vi "NT4 Prepare Tree Entries.vi"(11 "Topic List":T3(array[cluster]) {"NT_Type" items=["NT_Unassigned"=0, "NT_Boolean"=1, "NT_Double"=2, "NT_String"=4, "NT_Raw"=8, "NT_BooleanArray"=16, "NT_DoubleArray"=32, "NT_StringArray"=64, "NT_RPC"=128, "NT_Integer"=256, "NT_Float"=512, "NT_IntegerArray"=1024, "NT_FloatArray"=2048]}) -> (2 "Tokens":string[](array[string]), 3 "Sorted Tree Rows":T2(array[cluster]) {"NT_Type" items=["NT_Unassigned"=0, "NT_Boolean"=1, "NT_Double"=2, "NT_String"=4, "NT_Raw"=8, "NT_BooleanArray"=16, "NT_DoubleArray"=32, "NT_StringArray"=64, "NT_RPC"=128, "NT_Integer"=256, "NT_Float"=512, "NT_IntegerArray"=1024, "NT_FloatArray"=2048]})   [LabVIEW 2025]
uses:
  <vilib>/Rock Robotics/Network Tables/NT Datatype.ctl
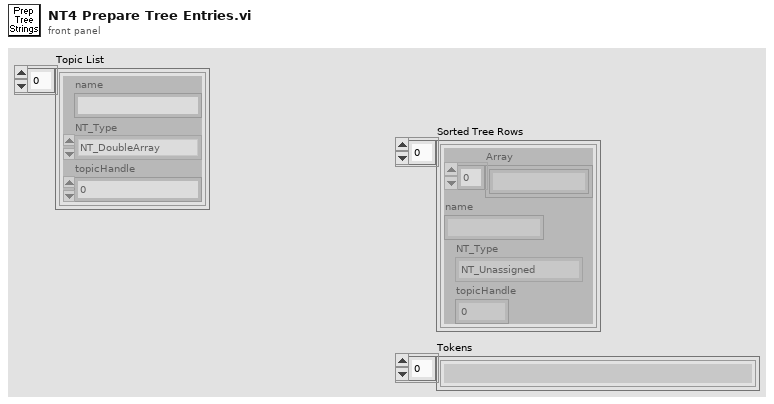
[diagram p1: front panel]
types:
  T1 = typedef "NT Datatype.ctl" = u32
  T2 = cluster{"Array":string[], "name":string, "NT_Type":T1, "topicHandle":u32}[]
  T3 = cluster{"name":string, "NT_Type":T1, "topicHandle":u32}[]
  T4 = cluster{"Array":string[], "name":string, "NT_Type":T1, "topicHandle":u32}
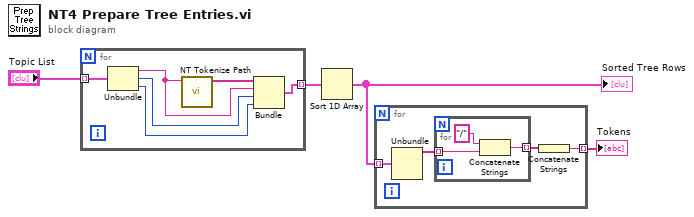
[diagram p0: block diagram]
diagram:
  n1 = for {
    tunnel: [w9] -> w4 mode=indexing
    tunnel: "Topic List" -> [w8] mode=indexing
    n2 = Unbundle(w8) -> ("name"=w7:string, "NT_Type"=w6:T1, "topicHandle"=w5:u32)
    n3 = call <vilib>:"NT Tokenize Path.vi"("Name"=w7) -> ("Array"=w10:string[])  [unwired: 10 in]
    n4 = Bundle("Array"=w10, "name"=w7, "NT_Type"=w6, "topicHandle"=w5) -> (w9:T4)  [unwired: 1 in]
  }
  n5 = Sort 1D Array(array=w4) -> (sorted array=w1:T2)
  "Sorted Tree Rows" <- w1
  n6 = for {
    tunnel: w1 -> [w14] mode=indexing
    tunnel: [w11] -> w3 mode=indexing
    n7 = Unbundle(w14) -> ("Array"=w13:string[])  [unwired: 3 out]
    n8 = for {
      tunnel: w13 -> [w16] mode=indexing
      tunnel: [w15] -> w12 mode=indexing
      n9 = Concatenate Strings("/", w16) -> (w15:string)
    }
    n10 = Concatenate Strings(w12) -> (w11:string)
  }
  "Tokens" <- w3
